vi "Constructor.vi"(11 "Dark Roast in":refnum<class "Dark Roast.lvclass">) -> (3 "Dark Roast out":refnum<class "Dark Roast.lvclass">)   [LabVIEW 2011, in "Dark Roast.lvclass"]
uses:
  Dark Roast.lvclass
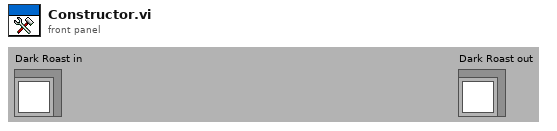
[diagram p1: front panel]
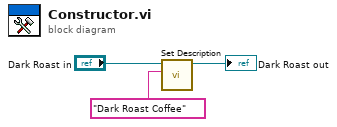
[diagram p0: block diagram]
diagram:
  n1 = call-dynamic "Set Description.vi"("Description"="Dark Roast Coffee", "Beverage in"="Dark Roast in") -> ("Beverage out"=→"Dark Roast out":refnum<class "Dark Roast.lvclass">)  [unwired: 9 in]
